vi "Send Value Change.vi"(5 "Use Label Text (F=Use Caption)":bool, 6 "Name (Get Text From Control)":string, 7 "Ctl Refnum":refnum<vi>, 8 "New Value":variant, 9 "Old Value":variant, 10 "Time":u32, 11 "Message Enqueuer in":refnum<class "Message Enqueuer.lvclass">) -> (0 "error out":errorcluster)   [LabVIEW 2015, in "ActorAutoRegistration.lvlib" / "ValueChangeMsg.lvclass"]
uses:
  ValueChangeMsg.lvclass
  <vilib>/ActorFramework/Message Enqueuer/Message Enqueuer.lvclass
  ValueChangeMsg.lvclass/ValueChangeMsg.ctl
  EventDataMessage/EventDataMessage.lvclass
panel:
  in  "error in (no error)":errorcluster
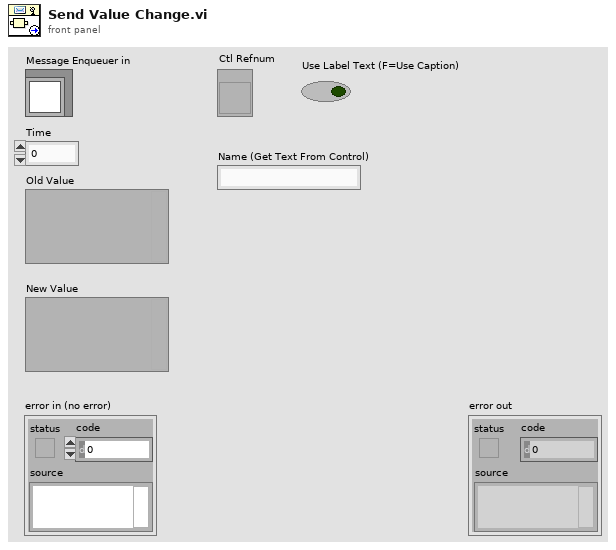
[diagram p1: front panel]
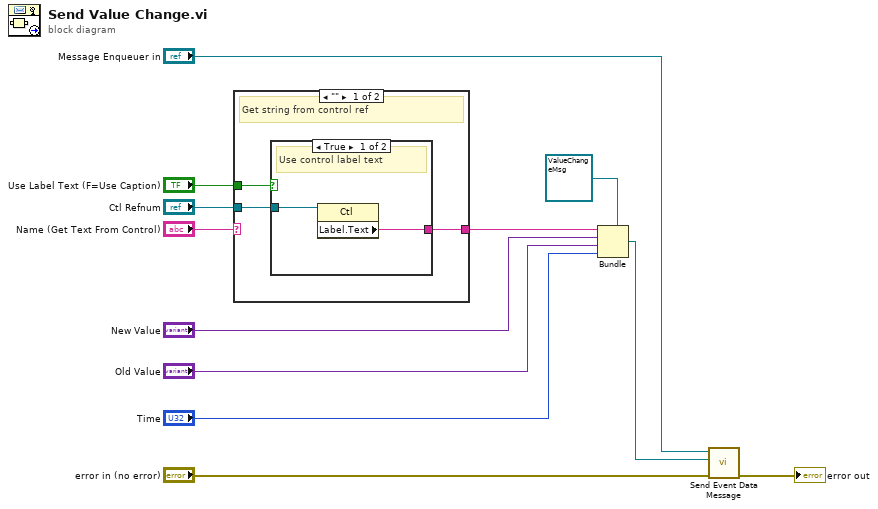
[diagram p0: block diagram]
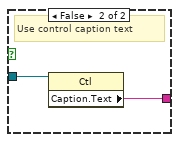
[diagram p2: hidden frame]
diagram:
  n1 = case shown="\"\"" "Name (Get Text From Control)" {
    selector: "Name (Get Text From Control)" -> [_ w20]
    tunnel: [w13 w20] -> w3
    tunnel: "Use Label Text (F=Use Caption)" -> [w15 _]
    tunnel: "Ctl Refnum" -> [w14 _]
    frame "" {
      # "Get string from control ref"
      n2 = case shown="True" w15 {
        tunnel: w14 -> [w17 w19]
        tunnel: [w16 w18] -> w13
        frame True {
          # "Use control label text"
          n3 = property class="Ctl"(reference=w17) -> ("Label.Text"=w16:string)  [unwired: 1 in, 2 out]
        }
        frame False {
          # "Use control caption text"
          n4 = property class="Ctl"(reference=w19) -> ("Caption.Text"=w18:string)  [unwired: 1 in, 2 out]
        }
      }
    }
    frame Default {
      # "Use string wired to input terminal"
    }
  }
  n5 = Bundle(cluster=refnum<class "ValueChangeMsg.lvclass"> refnum ("VariantValueMsg"), w3, "New Value", "Old Value", "Time") -> (w8:refnum<class "ValueChangeMsg.lvclass">)
  n6 = call "Send Event Data Message.vi"("error in (no error)"="error in (no error)", "EventDataMessage in"=w8, "Message Enqueuer in"="Message Enqueuer in") -> ("error out"=→"error out":errorcluster)  [unwired: 8 in]
